vi "XMLtoCalibration.vi"(0 "XML File Path":path) -> (2 "Calibrations":T1 {"Offset (V)" format="%_6p"; "Gain" format="%_6p"})   [LabVIEW 2018]
uses:
  Calibrations.ctl
  <vilib>/Utility/xml.llb/Read From XML File(string).vi
panel:
  in  "Calibrations proto":T1=[{"Gain"=0.0, "Offset (V)"=0.0, "Name"=""}] {"Offset (V)" format="%_6p"; "Gain" format="%_6p"}
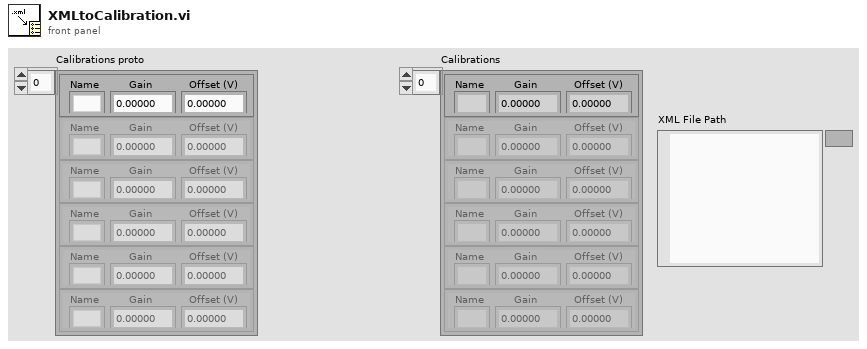
[diagram p1: front panel]
types:
  T1 = typedef "Calibrations.ctl" = cluster{"Gain":dbl, "Offset (V)":dbl, "Name":string}[]
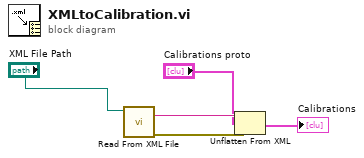
[diagram p0: block diagram]
diagram:
  n1 = call-poly <vilib>:"Read From XML File.vi"("XML File Path"="XML File Path") -> ("error out"=w3:errorcluster, "XML Elements"=w4:string)  [unwired: 8 in, 1 out]
  n2 = Unflatten From XML(xml string=w4, type="Calibrations proto", error in (no error)=w3) -> (value=→"Calibrations":T1)  [unwired: 1 out]
